vi "Bomb.vi"() -> ()   [LabVIEW 2014]
panel:
  out "Boolean 24":bool
  out "Boolean 23":bool
  out "Boolean 22":bool
  out "Boolean 21":bool
  out "Boolean 20":bool
  out "Boolean 19":bool
  out "Boolean 18":bool
  out "Boolean 17":bool
  in  "Boolean 16":bool
  in  "Boolean 15":bool
  in  "Boolean 14":bool
  in  "Boolean 13":bool
  in  "Boolean 12":bool
  in  "Boolean 11":bool
  in  "Boolean 10":bool
  in  "Boolean 9":bool
  out "Boolean 8":bool
  out "Boolean 7":bool
  out "Boolean 6":bool
  out "Boolean 5":bool
  out "Boolean 4":bool
  out "Boolean 3":bool
  out "Boolean 2":bool
  out "Boolean":bool
  in  "stop":bool
  out "Estado No.:":dbl
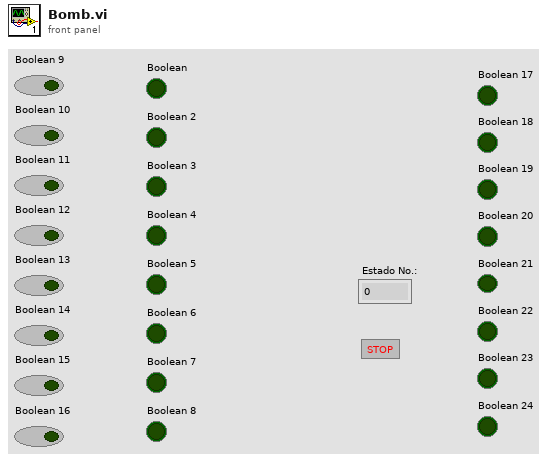
[diagram p1: front panel]
types:
  T1 = enum16{"D1", "D2", "D3", "D4", "D5", "D6", "D7", "D8"}
  T2 = enum16{"E1", "E2", "E3", "E4", "E5", "E6", "E7", "E8"}
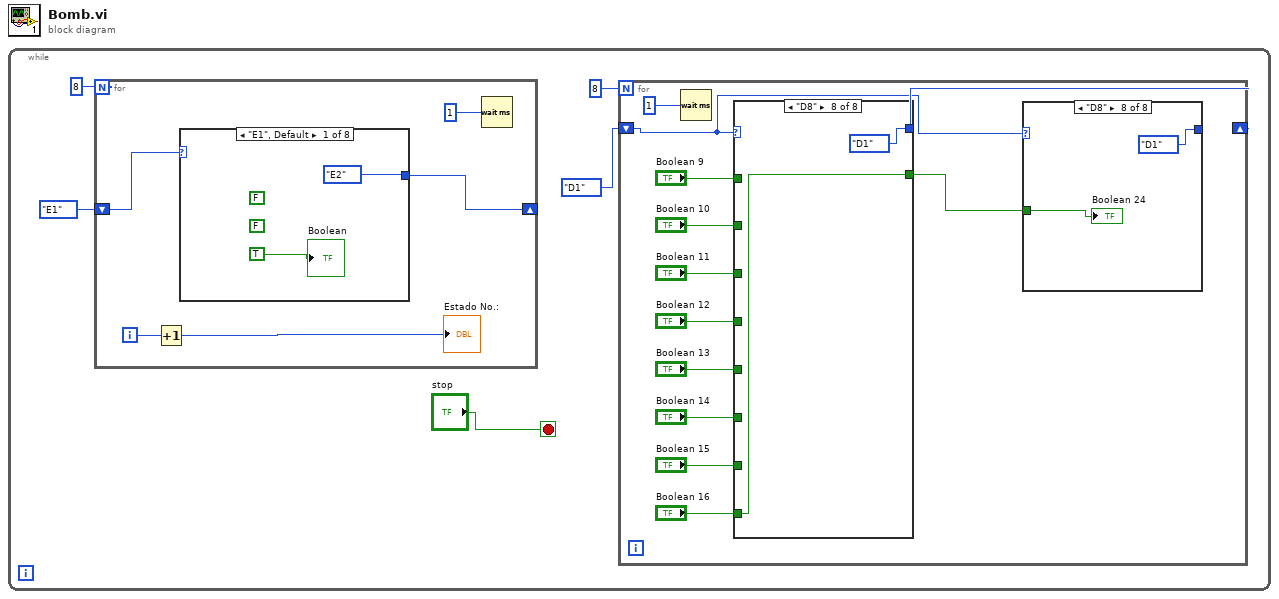
[diagram p0: block diagram]
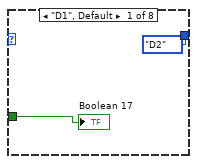
[diagram p2: hidden frame]
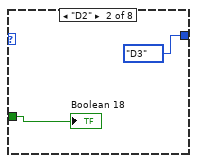
[diagram p3: hidden frame]
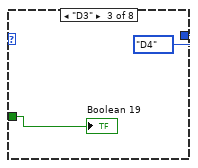
[diagram p4: hidden frame]
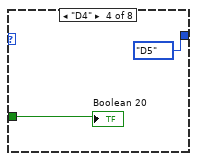
[diagram p5: hidden frame]
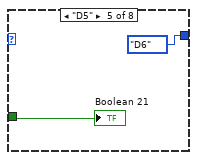
[diagram p6: hidden frame]
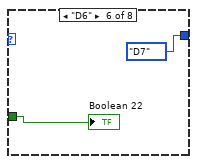
[diagram p7: hidden frame]
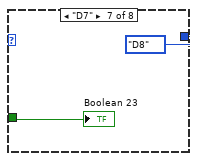
[diagram p8: hidden frame]
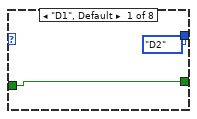
[diagram p9: hidden frame]
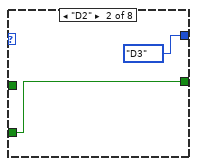
[diagram p10: hidden frame]
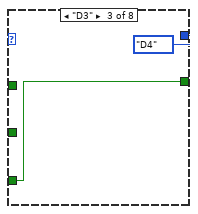
[diagram p11: hidden frame]
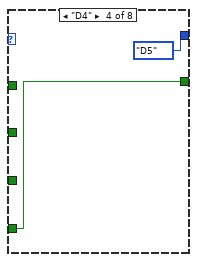
[diagram p12: hidden frame]
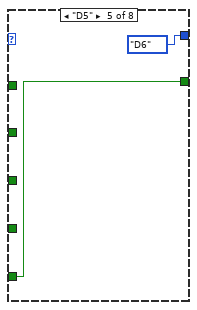
[diagram p13: hidden frame]
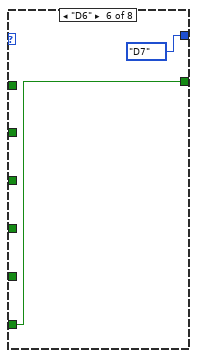
[diagram p14: hidden frame]
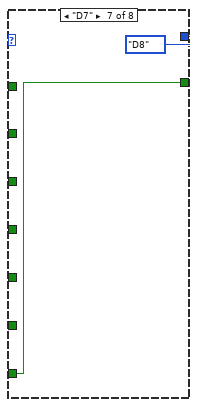
[diagram p15: hidden frame]
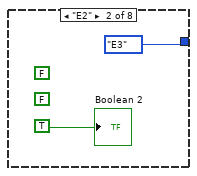
[diagram p16: hidden frame]
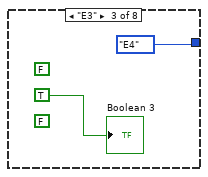
[diagram p17: hidden frame]
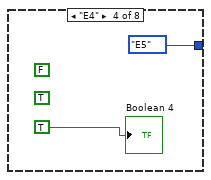
[diagram p18: hidden frame]
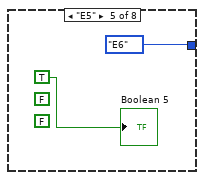
[diagram p19: hidden frame]
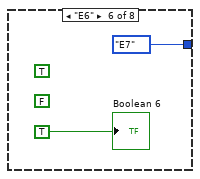
[diagram p20: hidden frame]
diagram:
  n1 = while {
    stop <- "stop" stop-if-true
    n2 = for {
      N: 8 -> [_]
      shift-right: [w50] -> _
      shift-left: T2."E1" -> [w51]
      i -> [w52]
      n3 = Increment(x=w52) -> (x+1=→"Estado No.:":i32)
      n4 = case shown="\"E1\", Default" w51 {
        tunnel: [T2."E2" T2."E3" T2."E4" T2."E5" T2."E6" T2."E7" T2."E8" T2."E1"] -> w50
        frame "E1", Default {
          (unwired) FALSE
          (unwired) FALSE
          "Boolean" <- TRUE
        }
        frame "E2" {
          (unwired) FALSE
          (unwired) FALSE
          "Boolean 2" <- TRUE
        }
        frame "E3" {
          (unwired) FALSE
          (unwired) FALSE
          "Boolean 3" <- TRUE
        }
        frame "E4" {
          (unwired) TRUE
          (unwired) FALSE
          "Boolean 4" <- TRUE
        }
        frame "E5" {
          (unwired) FALSE
          (unwired) FALSE
          "Boolean 5" <- TRUE
        }
        frame "E6" {
          (unwired) FALSE
          (unwired) TRUE
          "Boolean 6" <- TRUE
        }
        frame "E7" {
          (unwired) FALSE
          (unwired) TRUE
          "Boolean 7" <- TRUE
        }
        frame "E8" {
          (unwired) TRUE
          (unwired) TRUE
          "Boolean 8" <- TRUE
        }
      }
      n5 = Wait (ms)(milliseconds to wait=1) -> ()  [unwired: 1 out]
    }
    n6 = for {
      N: 8 -> [_]
      shift-right: [w9] -> _
      shift-left: T1."D1" -> [w7]
      n7 = Wait (ms)(milliseconds to wait=1) -> ()  [unwired: 1 out]
      n8 = case shown="\"D8\"" w7 {
        tunnel: "Boolean 9" -> [w35 _ _ _ _ _ _ _]
        tunnel: "Boolean 10" -> [_ w37 _ _ _ _ _ _]
        tunnel: "Boolean 11" -> [_ _ w39 _ _ _ _ _]
        tunnel: "Boolean 12" -> [_ _ _ w41 _ _ _ _]
        tunnel: "Boolean 13" -> [_ _ _ _ w43 _ _ _]
        tunnel: "Boolean 14" -> [_ _ _ _ _ w45 _ _]
        tunnel: "Boolean 15" -> [_ _ _ _ _ _ w47 _]
        tunnel: "Boolean 16" -> [_ _ _ _ _ _ _ w49]
        tunnel: [w35 w37 w39 w41 w43 w45 w47 w49] -> w6
        tunnel: [T1."D2" T1."D3" T1."D4" T1."D5" T1."D6" T1."D7" T1."D8" T1."D1"] -> w9
        frame "D1", Default {
        }
        frame "D2" {
        }
        frame "D3" {
        }
        frame "D4" {
        }
        frame "D5" {
        }
        frame "D6" {
        }
        frame "D7" {
        }
        frame "D8" {
        }
      }
      n9 = case shown="\"D8\"" w7 {
        tunnel: [T1."D2" T1."D3" T1."D4" T1."D5" T1."D6" T1."D7" T1."D8" T1."D1"] -> _
        tunnel: w6 -> [w18 w20 w22 w24 w26 w28 w30 w32]
        frame "D1", Default {
          "Boolean 17" <- w18
        }
        frame "D2" {
          "Boolean 18" <- w20
        }
        frame "D3" {
          "Boolean 19" <- w22
        }
        frame "D4" {
          "Boolean 20" <- w24
        }
        frame "D5" {
          "Boolean 21" <- w26
        }
        frame "D6" {
          "Boolean 22" <- w28
        }
        frame "D7" {
          "Boolean 23" <- w30
        }
        frame "D8" {
          "Boolean 24" <- w32
        }
      }
    }
  }
